vi "Set Report Header Text.vi"(0 "report in":refnum<class "NI_HTML.lvclass">, 5 "left header text":string, 7 "center header text":string, 9 "right header text":string, 11 "error in (no error)":errorcluster, 12 "HTML header size":enum16{"H1", "H2", "H3", "H4", "H5", "H6", "H7"}(ring)=enum."H3", 13 "header placement":enum16{"Top of Document", "Append to Body"}(ring)) -> (4 "report out":refnum<class "NI_HTML.lvclass">, 15 "error out":errorcluster)   [LabVIEW 2017, in "NI_HTML.lvclass"]
doc: "Sets the text of the report header."
uses:
  <vilib>/Utility/NIReport.llb/HTML/NI_HTML.lvclass
  <vilib>/Utility/NIReport.llb/HTML/NI_HTML.lvclass/NI_HTML.ctl
  <vilib>/Utility/NIReport.llb/NI_ReportGenerationCore.lvlib
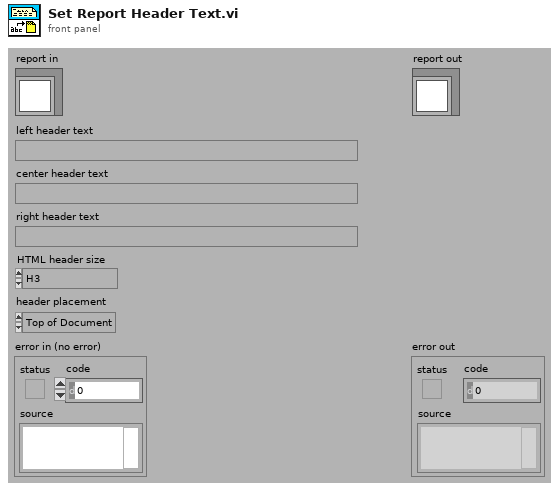
[diagram p1: front panel]
types:
  T1 = typedef "NI_ReportGenerationCore.lvlib/HTML Report Data.ctl" = cluster{"Body Text":string, "Font Tag":string, "Title Text":string, "Header Text":string, "Footer Text":string, "Image List":path[]}
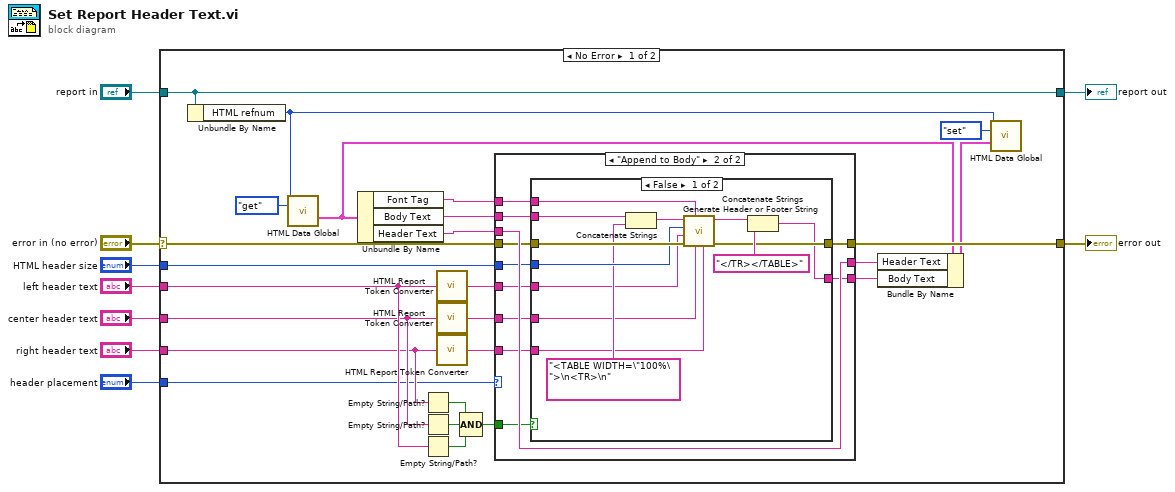
[diagram p0: block diagram]
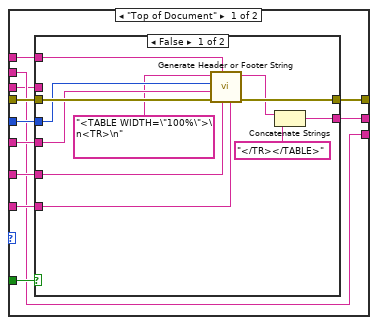
[diagram p2: hidden frame]
diagram:
  n1 = case shown="No Error" "error in (no error)" {
    selector: "error in (no error)" -> [w17 w85]
    tunnel: [w16 w85] -> w8
    tunnel: [w11 w84] -> w6
    tunnel: "report in" -> [w11 w84]
    tunnel: "HTML header size" -> [w22 _]
    tunnel: "left header text" -> [w21 _]
    tunnel: "center header text" -> [w20 _]
    tunnel: "right header text" -> [w19 _]
    tunnel: "header placement" -> [w18 _]
    frame No Error {
      n2 = Unbundle By Name(w11) -> ("HTML refnum"=w10:u32)
      n3 = call <vilib>:"HTML Data Global.vi"("HTML refnum"=w10, "menu"=enum16{"init", "get", "set", "delete"}."get") -> ("HTML report data out"=w12:T1)  [unwired: 1 in, 12 out]
      n4 = Unbundle By Name(w12) -> ("Font Tag"=w24:string, "Body Text"=w27:string, "Header Text"=w26:string)
      n5 = Empty String/Path?(string/path=w19) -> (empty?=w28:bool)
      n6 = Empty String/Path?(string/path=w20) -> (empty?=w29:bool)
      n7 = Empty String/Path?(string/path=w21) -> (empty?=w30:bool)
      n8 = call <vilib>:"HTML Report Token Converter.vi"("String In"=w21) -> ("String Out"=w32:string)
      n9 = call <vilib>:"HTML Report Token Converter.vi"("String In"=w20) -> ("String Out"=w33:string)
      n10 = call <vilib>:"HTML Report Token Converter.vi"("String In"=w19) -> ("String Out"=w34:string)
      n11 = Compound Arithmetic op=AND(w28, w29, w30) -> (w31:bool)
      n12 = case shown="\"Append to Body\"" w18 {
        tunnel: w31 -> [w44 w63]
        tunnel: w32 -> [w42 w67]
        tunnel: w33 -> [w43 w65]
        tunnel: w34 -> [w45 w64]
        tunnel: w17 -> [w40 w60]
        tunnel: [w37 w68] -> w23
        tunnel: [w38 w61] -> w16
        tunnel: w24 -> [w39 w58]
        tunnel: w22 -> [w41 w66]
        tunnel: [w36 w62] -> w25
        tunnel: w26 -> [w35 w68]
        tunnel: w27 -> [w36 w59]
        frame "Top of Document" {
          n13 = case shown="False" w44 {
            tunnel: w42 -> [w50 _]
            tunnel: w43 -> [w49 _]
            tunnel: w45 -> [w48 _]
            tunnel: [w53 w57] -> w38
            tunnel: w40 -> [w54 w57]
            tunnel: w39 -> [w52 _]
            tunnel: w41 -> [w51 _]
            tunnel: [w56 _] -> w37
            tunnel: w35 -> [_ _]
            frame False {
              n14 = call <vilib>:"Generate Header or Footer String.vi"("Right Text"=w48, "Center Text"=w49, "Font Tag"=w52, "error in (no error)"=w54, "Left Text"=w50, "size"=w51, "HTML in"="<TABLE WIDTH=\"100%\">\n<TR>\n" ("Substring")) -> ("error out"=w53:errorcluster, "HTML out"=w47:string)  [unwired: 3 out]
              n15 = Concatenate Strings(w47, "</TR></TABLE>" ("Substring")) -> (w56:string)
            }
            frame True {
            }
          }
        }
        frame "Append to Body" {
          n16 = case shown="False" w63 {
            tunnel: w67 -> [w74 _]
            tunnel: w65 -> [w73 _]
            tunnel: w64 -> [w72 _]
            tunnel: [w71 w83] -> w61
            tunnel: w60 -> [w81 w83]
            tunnel: w59 -> [w77 w82]
            tunnel: w66 -> [w80 _]
            tunnel: [w69 w82] -> w62
            tunnel: w58 -> [w70 _]
            frame False {
              n17 = Concatenate Strings(w77, "<TABLE WIDTH=\"100%\">\n<TR>\n" ("Substring")) -> (w76:string)
              n18 = call <vilib>:"Generate Header or Footer String.vi"("Right Text"=w72, "Center Text"=w73, "Font Tag"=w70, "error in (no error)"=w81, "Left Text"=w74, "size"=w80, "HTML in"=w76) -> ("error out"=w71:errorcluster, "HTML out"=w79:string)  [unwired: 3 out]
              n19 = Concatenate Strings(w79, "</TR></TABLE>" ("Substring")) -> (w69:string)
            }
            frame True {
            }
          }
        }
      }
      n20 = Bundle By Name(cluster=w12, "Header Text"=w23, "Body Text"=w25) -> (w13:T1)
      n21 = call <vilib>:"HTML Data Global.vi"("HTML refnum"=w10, "menu"=enum16{"init", "get", "set", "delete"}."set", "HTML report data in"=w13) -> ()  [unwired: 13 out]
    }
    frame Error {
    }
  }
  "error out" <- w8
  "report out" <- w6
